vi "Simulation Console.vi"() -> ()   [LabVIEW 2012]
doc: "[Covers: UI1]"
uses:
  DataType/Simulation Console_User Action.ctl
  DataType/Simulation Console_Data From UI.ctl
  DataType/Simulation Console_Controller Command.ctl
  DataType/Simulation Console_Command To UI.ctl
  DataType/FGV_Message Manager_Command.ctl
  Controls/Keypad.xctl
panel:
  in  "Keypad":u32(xcontrol)
  out "ATM Messages":string
  out "Right Menu 3":string
  out "Right Menu 2":string
  out "Right Menu 1":string
  out "Left Menu 3":string
  out "Left Menu 2":string
  out "Left Menu 1":string
  in  "Right Button 3":bool
  in  "Right Button 2":bool
  in  "Right Button 1":bool
  in  "Left Button 3":bool
  in  "Left Button 2":bool
  in  "Left Button 1":bool
  in  "Card Slot":bool
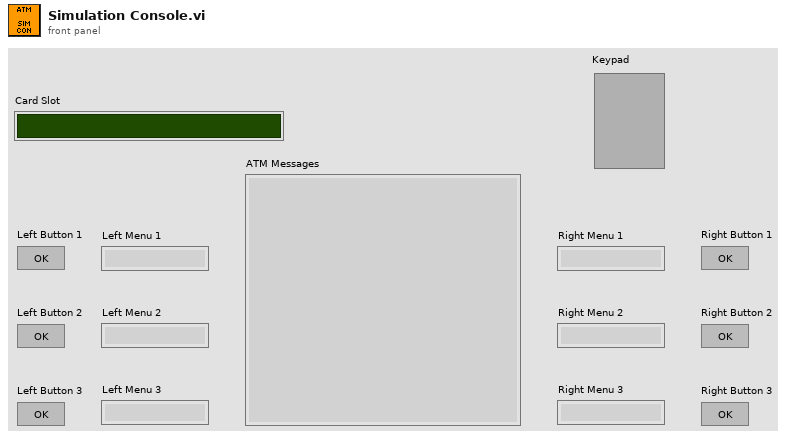
[diagram p1: front panel]
types:
  T1 = typedef "FGV_Message Manager_Command.ctl" = enum16{"Initial", "Close", "SendMessage", "SendButton", "DisableUI", "ClearKeypad", "ReturnCard", "RecieveUserInput"}
  T2 = typedef "Simulation Console_Command To UI.ctl" = cluster{"Command":T3, "Parameter":variant}
  T3 = typedef "Simulation Console_Controller Command.ctl" = enum16{"Show Message", "Return Card", "Stop", "Show Menu", "Clear Keypad", "Disable UI Element"}
  T4 = typedef "Simulation Console_Data From UI.ctl" = cluster{"UI to Controller Message":T5, "Parameter":variant}
  T5 = typedef "Simulation Console_User Action.ctl" = enum16{"Button Press", "Card Insert", "Card Remove", "Keypad Input"}
  T6 = enum8{"Enabled", "Disabled", "Disabled and Grayed Out"}
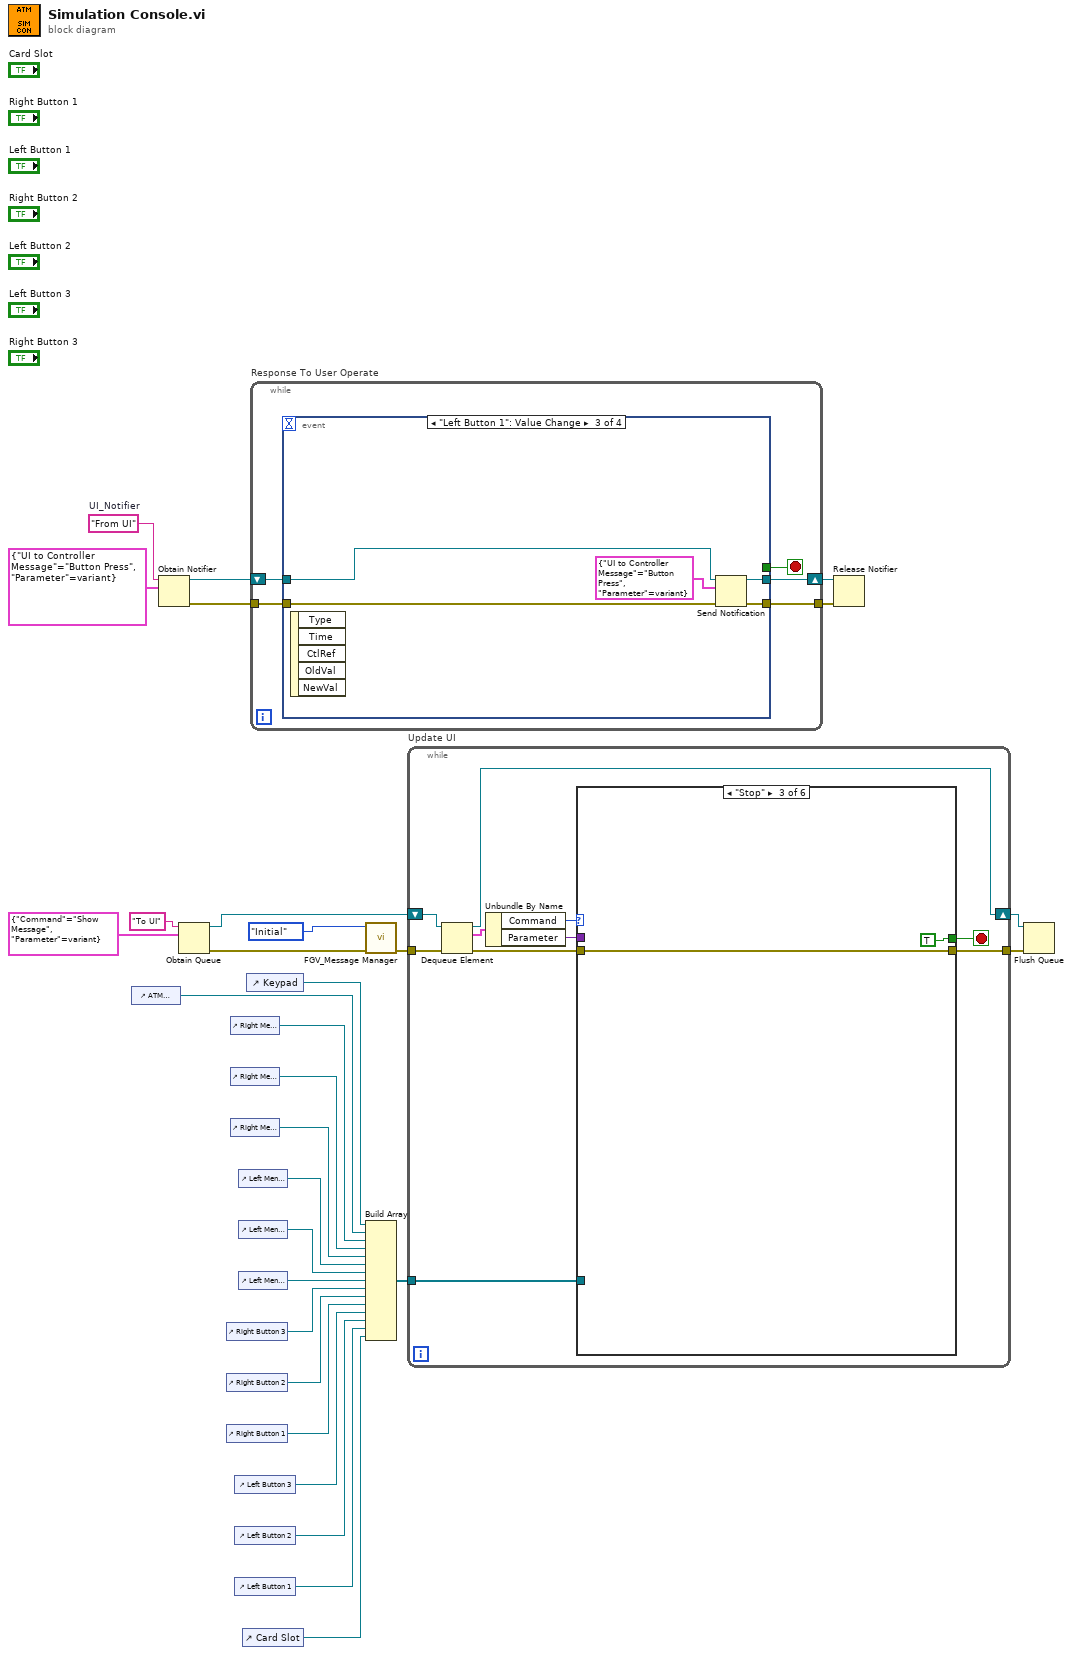
[diagram p0: block diagram]
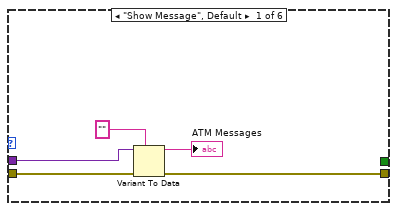
[diagram p2: hidden frame]
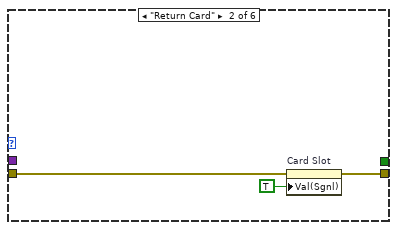
[diagram p3: hidden frame]
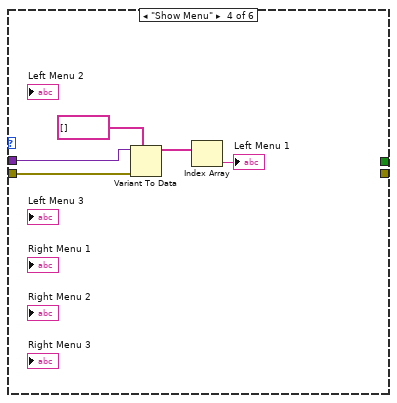
[diagram p4: hidden frame]
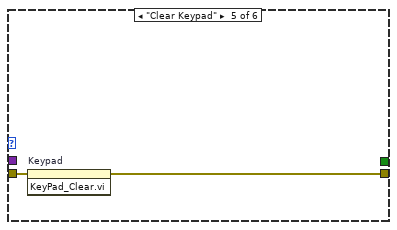
[diagram p5: hidden frame]
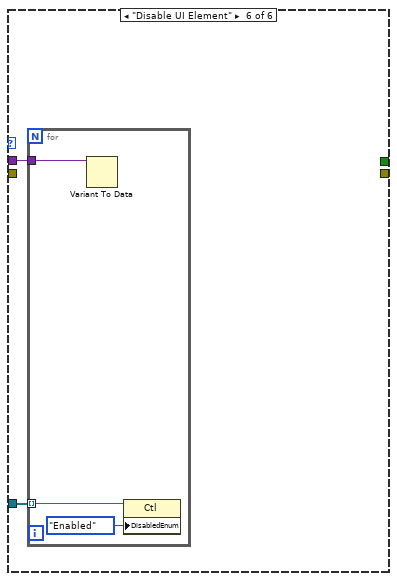
[diagram p6: hidden frame]
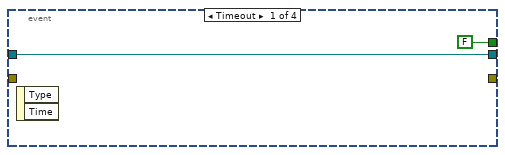
[diagram p7: hidden frame]
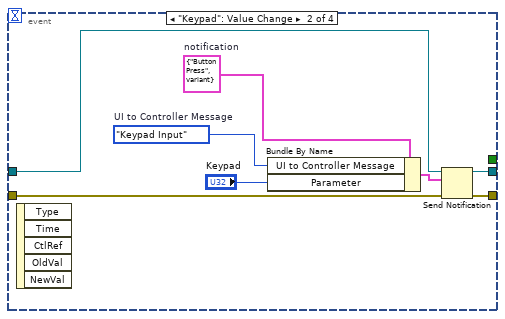
[diagram p8: hidden frame]
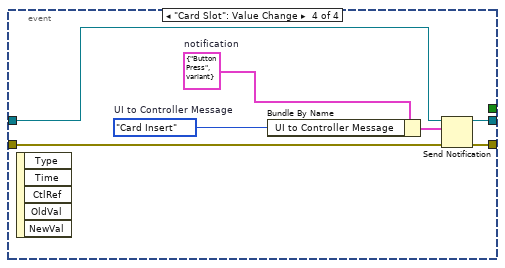
[diagram p9: hidden frame]
diagram:
  w30 = "From UI"  # UI_Notifier
  n1 = control-ref of="ATM Messages"() -> (w15:refnum<vi>)
  n2 = Obtain Notifier(name (unnamed)=w30, notification data type=T4 {"UI to Controller Message"=enum."Button Press", "Parameter"=variant}) -> (notifier out=w29:refnum<notifier>, error out=w18:errorcluster)  [unwired: 2 in, 1 out]
  n3 = Obtain Queue(name (unnamed)="To UI", element data type=T2 {"Command"=enum."Show Message", "Parameter"=variant}) -> (queue out=w26:refnum<queue>, error out=w21:errorcluster)  [unwired: 3 in, 1 out]
  n4 = control-ref of="Right Button 3"() -> (w8:refnum<vi>)
  n5 = control-ref of="Right Button 2"() -> (w7:refnum<vi>)
  n6 = control-ref of="Right Button 1"() -> (w6:refnum<vi>)
  n7 = control-ref of="Right Menu 3"() -> (w14:refnum<vi>)
  n8 = control-ref of="Right Menu 2"() -> (w13:refnum<vi>)
  n9 = control-ref of="Right Menu 1"() -> (w12:refnum<vi>)
  n10 = control-ref of="Left Button 3"() -> (w5:refnum<vi>)
  n11 = control-ref of="Left Button 2"() -> (w4:refnum<vi>)
  n12 = control-ref of="Left Button 1"() -> (w3:refnum<vi>)
  n13 = control-ref of="Left Menu 3"() -> (w11:refnum<vi>)
  n14 = control-ref of="Left Menu 2"() -> (w10:refnum<vi>)
  n15 = control-ref of="Left Menu 1"() -> (w9:refnum<vi>)
  n16 = control-ref of="Card Slot"() -> (w2:refnum<vi>)
  n17 = control-ref of="Keypad"() -> (w16:refnum<vi>)
  n18 = while "Response To User Operate" {
    shift-right: [w33] -> w28
    shift-left: w29 -> [w34]
    tunnel: w18 -> [w32]
    tunnel: [w31] -> w17
    stop <- w35 stop-if-true
    n19 = event shown="[2] \"Left Button 1\": Value Change" {
      selector: _ -> [_ _ _ _]
      dyn-events: _ -> [_ _ _ _]
      timeout: _ -> [_ _ _ _]
      tunnel: [FALSE _ _ _] -> w35
      tunnel: w34 -> [w36 w45 w50 w57]
      tunnel: [w36 w44 w48 w56] -> w33
      tunnel: w32 -> [_ w39 w49 w51]
      tunnel: [_ w38 w47 w52] -> w31
      event Timeout {
        n20 = event-data() -> ()  [unwired: 1 in, 2 out]
      }
      event "Keypad": Value Change {
        w41 = Simulation_Console_User_Action."Keypad Input"  # UI to Controller Message
        w43 = T4 {"UI to Controller Message"=enum."Button Press", "Parameter"=variant}  # notification
        n21 = event-data() -> ()  [unwired: 1 in, 5 out]
        n22 = Bundle By Name(cluster=w43, "UI to Controller Message"=w41, "Parameter"="Keypad") -> (w42:T4)
        n23 = Send Notification(notification=w42, notifier=w45, error in (no error)=w39) -> (notifier out=w44:refnum<notifier>, error out=w38:errorcluster)
      }
      event "Left Button 1": Value Change {
        n24 = event-data() -> ()  [unwired: 1 in, 5 out]
        n25 = Send Notification(notification=T4 {"UI to Controller Message"=enum."Button Press", "Parameter"=variant}, notifier=w50, error in (no error)=w49) -> (notifier out=w48:refnum<notifier>, error out=w47:errorcluster)
      }
      event "Card Slot": Value Change {
        w53 = Simulation_Console_User_Action."Card Insert"  # UI to Controller Message
        w55 = T4 {"UI to Controller Message"=enum."Button Press", "Parameter"=variant}  # notification
        n26 = event-data() -> ()  [unwired: 1 in, 5 out]
        n27 = Bundle By Name(cluster=w55, "UI to Controller Message"=w53) -> (w54:T4)
        n28 = Send Notification(notification=w54, notifier=w57, error in (no error)=w51) -> (notifier out=w56:refnum<notifier>, error out=w52:errorcluster)
      }
    }
  }
  n29 = call "FGV_Message Manager.vi"("error in (no error)"=w21, "Command"=FGV_Message_Manager_Command."Initial") -> ("error out"=w20:errorcluster)  [unwired: 7 in, 2 out]
  n30 = Build Array(w16, w15, w14, w13, w12, w11, w10, w9, w8, w7, w6, w5, w4, w3, w2) -> (w1:refnum<vi>[])
  n31 = while "Update UI" {
    tunnel: w20 -> [w65]
    tunnel: [w60] -> w24
    shift-right: [w66] -> w25
    shift-left: w26 -> [w67]
    tunnel: w1 -> [w58]
    stop <- w59 stop-if-true
    n32 = Dequeue Element(queue=w67, error in (no error)=w65) -> (queue out=w66:refnum<queue>, element=w64:T2, error out=w61:errorcluster)  [unwired: 1 in, 1 out]
    n33 = Unbundle By Name(w64) -> ("Command"=w63:T3, "Parameter"=w62:variant)
    n34 = case shown="\"Stop\"" w63 {
      tunnel: w62 -> [w72 _ _ w82 _ w85]
      tunnel: w61 -> [w69 w74 w77 w78 w84 _]
      tunnel: [w68 w73 w77 _ w83 _] -> w60
      tunnel: [_ _ TRUE _ _ _] -> w59
      tunnel: w58 -> [_ _ _ _ _ w86]
      frame "Show Message", Default {
        n35 = Variant To Data(error in=w69, type="" ("ATM Messages"), Variant=w72) -> (data=→"ATM Messages":string, error out=w68:errorcluster)
      }
      frame "Return Card" {
        n36 = property on="Card Slot" class="Bool (strict)"(error in=w74, "Val(Sgnl)"=TRUE ("Value (Signaling)")) -> (error out=w73:errorcluster)  [unwired: 1 in, 1 out]
      }
      frame "Stop" {
      }
      frame "Show Menu" {
        n37 = Variant To Data(error in=w78, type=string[] [], Variant=w82) -> (data=w80:string[])  [unwired: 1 out]
        n38 = Index Array(array=w80) -> (element=→"Left Menu 1":string)  [unwired: 1 in]
      }
      frame "Clear Keypad" {
        n39 = invoke on="Keypad" class="Keypad (strict)" method="KeyPad_Clear.vi"(error in=w84) -> (error out=w83:errorcluster)  [unwired: 2 in, 2 out]
      }
      frame "Disable UI Element" {
        n40 = for {
          tunnel: w86 -> [w89] mode=indexing
          tunnel: w85 -> [w88]
          n41 = Variant To Data(Variant=w88) -> ()  [unwired: 2 in, 2 out]
          n42 = property class="Ctl"(reference=w89, "DisabledEnum"=T6."Enabled" ("Disabled")) -> ()  [unwired: 1 in, 2 out]
        }
      }
    }
  }
  n43 = Release Notifier(notifier=w28, error in (no error)=w17) -> ()  [unwired: 1 in, 3 out]
  n44 = Flush Queue(queue=w25, error in (no error)=w24) -> ()  [unwired: 3 out]
